vi "Stream Test EKG.vi"() -> ()   [LabVIEW 2015]
uses:
  <vilib>/DAQmx/write.llb/DAQmx Write (Analog 1D DBL 1Chan NSamp).vi
  <vilib>/DAQmx/create/channels.llb/DAQmx Create Channel (AO-Voltage-Basic).vi
  <vilib>/DAQmx/configure/timing.llb/DAQmx Timing (Sample Clock).vi
  <vilib>/DAQmx/miscellaneous.llb/DAQmx Fill In Error Info.vi
  <resource>/objmgr/daqmx.rc
panel:
  in  "stop":bool
  in  "Channel":tag="PXI1Slot3/ao0"
  out "Graph":dbl[](graph)
  in  "Path":path=path "C:/Data/XYZ DATA/ekg-1.f64"
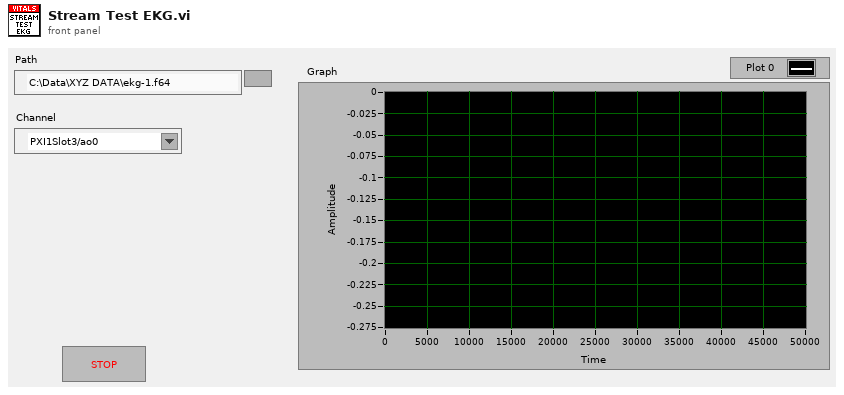
[diagram p1: front panel]
types:
  T1 = typedef "DL-File Header.ctl" = cluster{"path":path, "nchan":i32, "names":string[], "Fs (Hz)":dbl, "pts/read/ch":i32, "header size":i32, "nrecords":i32, "last read":i32, "bytes/read":i32}
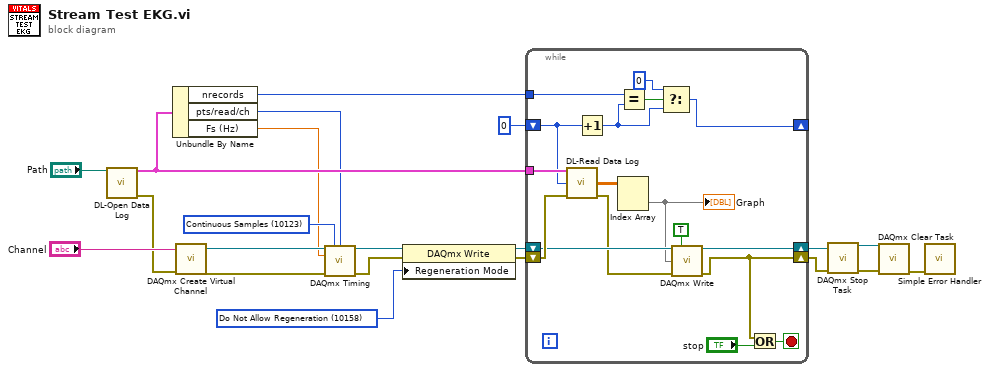
[diagram p0: block diagram]
diagram:
  w10 = 10158 items=["Allow Regeneration"=10097, "Do Not Allow Regeneration"=10158] ("RegenMode")
  w17 = 10123 items=["Finite Samples"=10178, "Continuous Samples"=10123, "Hardware Timed Single Point"=12522] ("sample mode")
  n1 = call "DL-Open Data Log.vi"("Path"="Path") -> ("Header"=w20:T1, "error out"=w18:errorcluster)  [unwired: 13 in]
  n2 = Unbundle By Name(w20) -> ("nrecords"=w9:i32, "pts/read/ch"=w13:i32, "Fs (Hz)"=w14:dbl)
  n3 = call-poly <vilib>:"DAQmx Create Virtual Channel.vi"("physical channels"="Channel", "error in"=w18) -> ("task out"=w15:refnum<k21>, "error out"=w16:errorcluster)  [unwired: 12 in]
  n4 = call-poly <vilib>:"DAQmx Timing.vi"("task/channels in"=w15, "sample mode"=w17, "samples per channel"=w13, "rate"=w14, "error in"=w16) -> ("task out"=w12:refnum<k21>, "error out"=w11:errorcluster)  [unwired: 9 in]
  n5 = property class="DAQmx Write"(reference=w12, error in=w11, "Regeneration Mode"=w10) -> (reference out=w6:refnum<k21>, error out=w7:errorcluster)
  n6 = while {
    tunnel: w20 -> [w38]
    tunnel: w9 -> [w26]
    shift-right: [w22] -> _
    shift-left: 0 -> [w27]
    shift-right: [w30] -> w5
    shift-left: w6 -> [w34]
    shift-right: [w28] -> w4
    shift-left: w7 -> [w35]
    stop <- w29 stop-if-true
    n7 = call "DL-Read Data Log.vi"("Header in"=w38, "First"=w27, "error in (no error)"=w35) -> ("Array"=w37:dbl[][], "error out"=w31:errorcluster)  [unwired: 10 in, 1 out]
    n8 = Increment(x=w27) -> (x+1=w24:i32)
    n9 = Index Array(array=w37) -> (element=w32:dbl[])  [unwired: 2 in]
    "Graph" <- w32
    n10 = Equal?(x=w26, y=w24) -> (x = y?=w25:bool)
    n11 = Select(t=0, s=w25, f=w24) -> (s? t:f=w22:i32)
    n12 = call-poly <vilib>:"DAQmx Write.vi"("task/channels in"=w34, "auto start"=TRUE, "data"=w32, "error in"=w31) -> ("task out"=w30:refnum<k21>, "error out"=w28:errorcluster)  [unwired: 9 in, 1 out]
    n13 = Or(x=w28, y="stop") -> (x .or. y?=w29:bool)
  }
  n14 = call <vilib>:"DAQmx Stop Task.vi"("task/channels in"=w5, "error in"=w4) -> ("task out"=w3:refnum<k21>, "error out"=w2:errorcluster)  [unwired: 12 in]
  n15 = call <vilib>:"DAQmx Clear Task.vi"("task in"=w3, "error in"=w2) -> ("error out"=w1:errorcluster)  [unwired: 13 in]
  n16 = call <vilib>:"Simple Error Handler.vi"("error in (no error)"=w1) -> ()  [unwired: 4 in, 5 out]
